vi "Flattening of SGL arrays.vi"() -> ()   [LabVIEW 2017]
uses:
  JSONtext.lvlib
panel:
  in  "Pretty Print?":bool
  in  "enable LabVIEW extensions?":bool=TRUE
  out "time":dbl format="%#_3p"
  out "JSON string":string
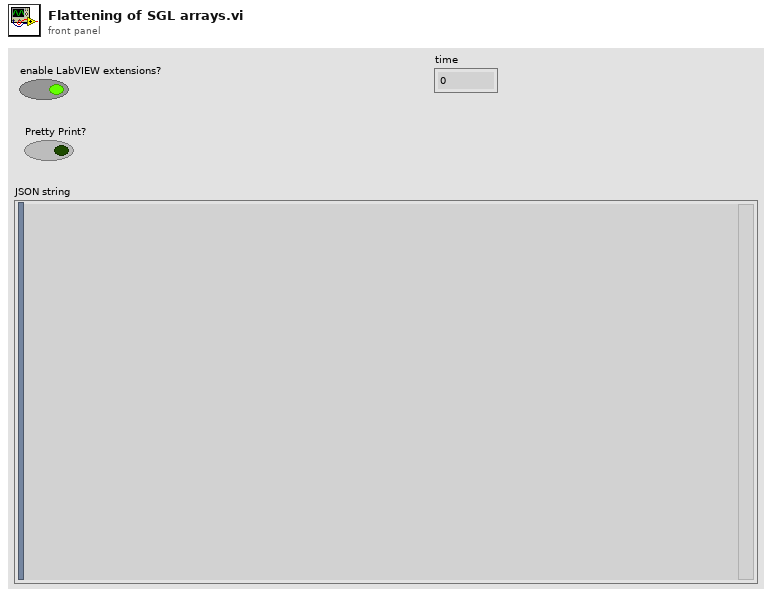
[diagram p1: front panel]
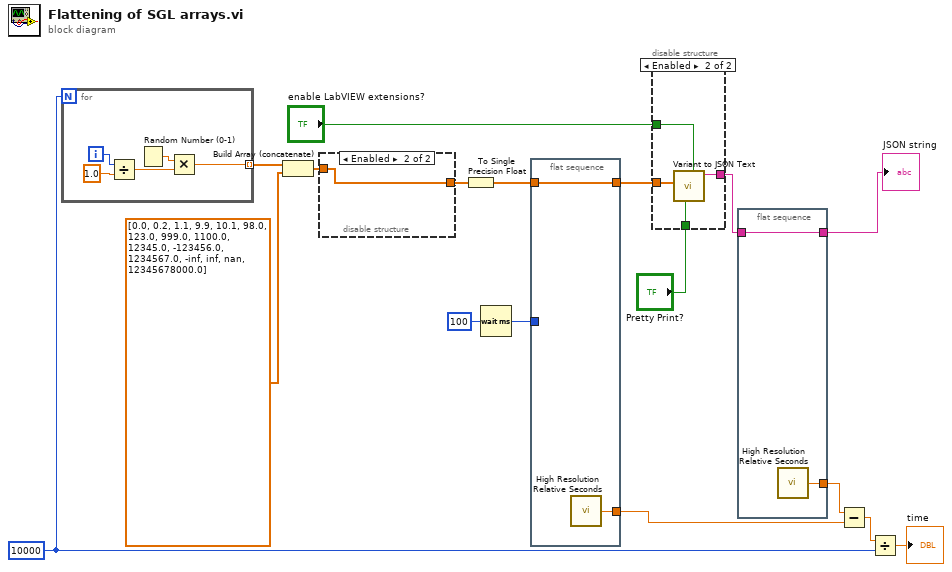
[diagram p0: block diagram]
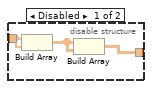
[diagram p2: hidden frame]
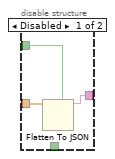
[diagram p3: hidden frame]
diagram:
  w10 = 10000
  n1 = for {
    N: w10 -> [_]
    tunnel: [w18] -> w14 mode=indexing
    i -> [w19]
    n2 = Divide(x=w19, y=1.0) -> (x/y=w21:dbl)
    n3 = Random Number (0-1)() -> (number: 0 to 1=w20:dbl)
    n4 = Multiply(x=w20, y=w21) -> (x*y=w18:dbl)
  }
  n5 = Build Array (concatenate)(w14, dbl[] [0.0, 0.2, 1.1, 9.9, 10.1, 98.0, 123.0, 999.0, 1100.0, 12345.0, -123456.0, 1234567.0, -inf, inf, nan, 12345678000.0]) -> (w2:dbl[])
  n6 = disable-structure shown="Enabled" {
    disable-tunnel: [w25 w26] -> w3
    disable-tunnel: w2 -> [w24 w26]
    frame Disabled {
      n7 = Build Array(w24, w24) -> (w23:dbl[][])
      n8 = Build Array(w23, w23) -> (w25:dbl[][][])
    }
    frame Enabled {
    }
  }
  n9 = To Single Precision Float(number=w3) -> (single precision float=w7:sgl[])
  n10 = Wait (ms)(milliseconds to wait=u32 100) -> (millisecond timer value=w5:u32)
  n11 = flat-sequence {
    tunnel: [w28] -> w15
    tunnel: w7 -> [w27]
    tunnel: [w27] -> w13
    tunnel: w5 -> [_]
    frame #0 {
      n12 = call <vilib>:"High Resolution Relative Seconds.vi"() -> ("relative seconds"=w28:dbl)
    }
  }
  n13 = disable-structure shown="Enabled" {
    disable-tunnel: [w31 w34] -> w17
    disable-tunnel: w13 -> [w30 w35]
    disable-tunnel: "enable LabVIEW extensions?" -> [w29 w33]
    disable-tunnel: "Pretty Print?" -> [_ w32]
    frame Disabled {
      n14 = Flatten To JSON(enable LabVIEW extensions? (T)=w29, anything=w30) -> (JSON string=w31:string)  [unwired: 1 in, 1 out]
    }
    frame Enabled {
      n15 = call "Variant to JSON Text.vi"("enable LabVIEW extensions? (T)"=w33, "Pretty Print?"=w32, "Variant"=w35) -> ("<JSON>"=w34:string)  [unwired: 6 in, 2 out]
    }
  }
  n16 = flat-sequence {
    tunnel: w17 -> [w36]
    tunnel: [w37] -> w16
    tunnel: [w36] -> w4
    frame #0 {
      n17 = call <vilib>:"High Resolution Relative Seconds.vi"() -> ("relative seconds"=w37:dbl)
    }
  }
  n18 = Subtract(x=w16, y=w15) -> (x-y=w12:dbl)
  n19 = Divide(x=w12, y=w10) -> (x/y=→"time":dbl)
  "JSON string" <- w4
